vi "GenerateTrajPoints.vi"(8 "Local Path":path=path "D:/Documents/LabVIEW Data/FRC_2019_OffseasC:/Users/Nick/Documents/LabVIEW Data/FRC_2019_Offseason_PathFollowing/PathFollowing/Paths", 9 "Use Local Path":bool=TRUE, 11 "CSV File Name":string="TestPath.csv") -> (2 "TrajectoryPointList":T1[](array[typedef]))   [LabVIEW 2018]
uses:
  MPTrajectoryPoint.ctl
  <vilib>/Utility/file.llb/Read Delimited Spreadsheet (DBL).vi
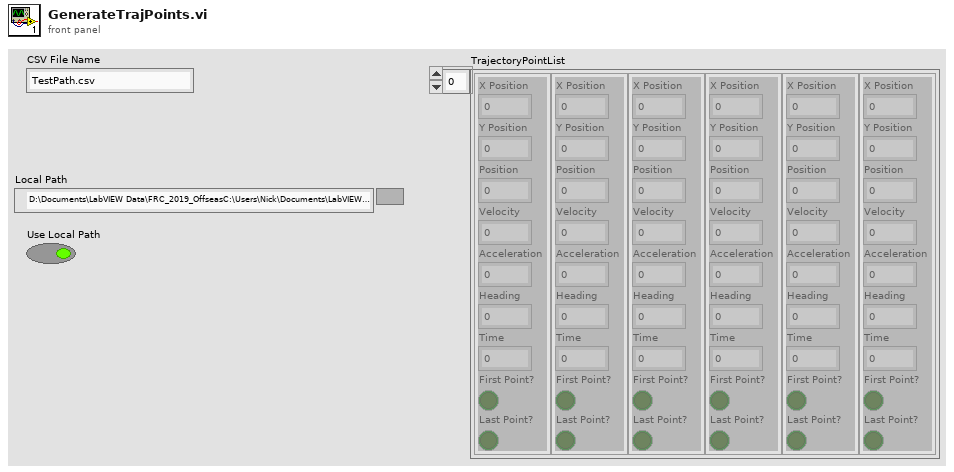
[diagram p1: front panel]
types:
  T1 = typedef "MPTrajectoryPoint.ctl" = cluster{"X Position":dbl, "Y Position":dbl, "Position":dbl, "Velocity":dbl, "Acceleration":dbl, "Heading":dbl, "Time":dbl, "First Point?":bool, "Last Point?":bool}
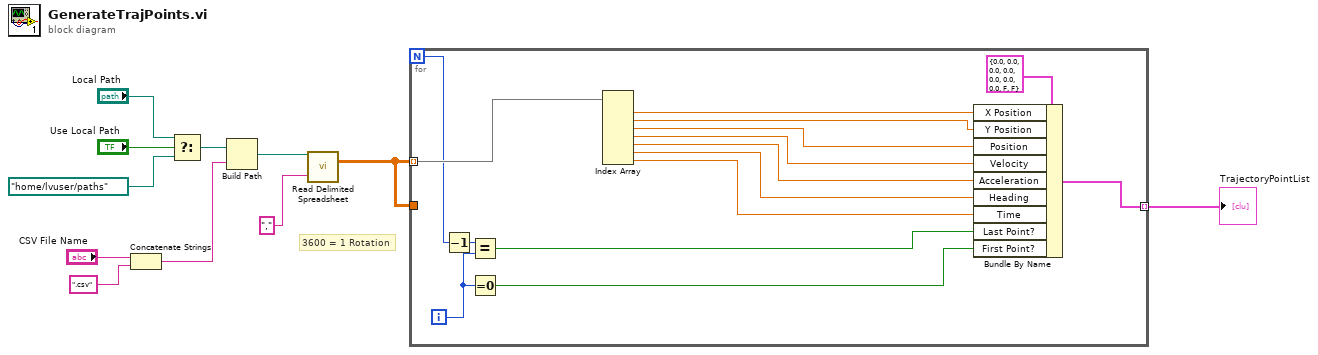
[diagram p0: block diagram]
diagram:
  # "3600 = 1 Rotation"
  n1 = Concatenate Strings("CSV File Name", ".csv") -> (w10:string)
  n2 = Select(t="Local Path", s="Use Local Path", f=path "/home/lvuser/paths" ("base path")) -> (s? t:f=w2:path)
  n3 = Build Path(base path=w2, name or relative path=w10) -> (appended path=w8:path)
  n4 = call-poly <vilib>:"Read Delimited Spreadsheet.vi"("file path (dialog if empty)"=w8, "delimiter (\\t)"="," ("delimiter (\\t)")) -> ("all rows"=w7:dbl[][])  [unwired: 8 in, 5 out]
  n5 = for {
    N -> [w25]
    tunnel: w7 -> [w26] mode=indexing
    tunnel: [w22] -> w1 mode=indexing
    tunnel: w7 -> [_]
    i -> [w24]
    n6 = Decrement(x=w25) -> (x-1=w23:i32)
    n7 = Equal?(x=w23, y=w24) -> (x = y?=w13:bool)
    n8 = Equal To 0?(x=w24) -> (x = 0?=w12:bool)
    n9 = Index Array(array=w26) -> (element #1=w20:dbl, element #2=w19:dbl, element #3=w18:dbl, element #4=w17:dbl, element #5=w16:dbl, element #6=w15:dbl, element #7=w14:dbl)  [unwired: 7 in]
    n10 = Bundle By Name(cluster=T1 {"X Position"=0.0, "Y Position"=0.0, "Position"=0.0, "Velocity"=0.0, "Acceleration"=0.0, "Heading"=0.0, "Time"=0.0, "First Point?"=FALSE, "Last Point?"=FALSE} ("MPTrajectoryPoint"), "X Position"=w20, "Y Position"=w19, "Position"=w18, "Velocity"=w17, "Acceleration"=w16, "Heading"=w15, "Time"=w14, "Last Point?"=w13, "First Point?"=w12) -> (w22:T1)
  }
  "TrajectoryPointList" <- w1
